vi "GCMPlugin_IsSupportingItem.vi"(8 "error in (no error)":errorcluster, 9 "VI Reference":refnum<vi>, 10 "ProjectItem Refnum":refnum<vi>, 11 "_ClassFieldsEditor in":refnum<class "_ClassFieldsEditor.lvclass">) -> (0 "error out":errorcluster, 2 "IsSupportingItem":bool, 3 "_ClassFieldsEditor out":refnum<class "_ClassFieldsEditor.lvclass">)   [LabVIEW 2014, in "_ClassFieldsEditor.lvclass"]
uses:
  _ClassFieldsEditor.lvclass
  GCMCore/Providers/Veritech_GCM/Support/Utilites/_ProjectItemsUtilities/_ProjectItemsUtilities.lvlib
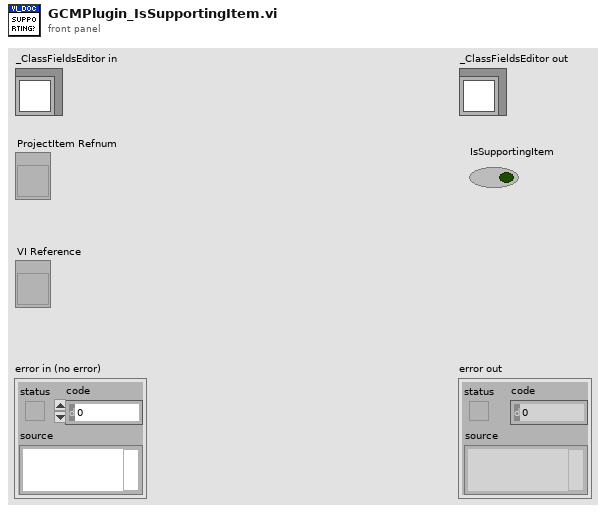
[diagram p1: front panel]
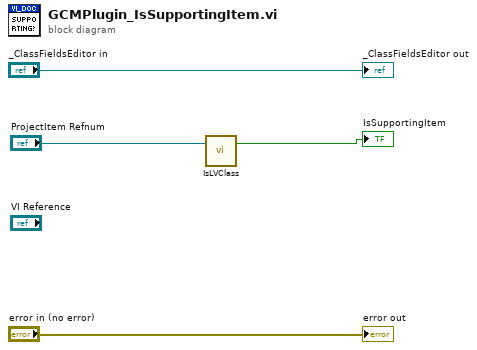
[diagram p0: block diagram]
diagram:
  n1 = call "IsLVClass.vi"("ProjectItem Refnum"="ProjectItem Refnum") -> ("IsLVClass?"=→"IsSupportingItem":bool)  [unwired: 2 in]
  "error out" <- "error in (no error)"
  "_ClassFieldsEditor out" <- "_ClassFieldsEditor in"
